vi "Send Perform Action on Target.vi"(7 "Message Priority (Normal)":T1=enum."Normal", 8 "error in":errorcluster, 9 "Point dent":string, 10 "Input":variant, 11 "Message Enqueuer":refnum<class "Message Enqueuer.lvclass">) -> (0 "error out":errorcluster, 2 "Output":variant, 3 "Message Enqueuer out":refnum<class "Message Enqueuer.lvclass">)   [LabVIEW 2023, in "IStudy Actor.lvlib" / "Perform Action on Target Msg.lvclass"]
doc: "This VI sends the message to an actor."
uses:
  Perform Action on Target Msg.lvclass
  Perform Action on Target Msg.lvclass/Perform Action on Target Msg.ctl
  DS-Reply-Msg/DS Reply Msg/DS Reply Msg.lvclass
  D:/git/DS-Reply-Msg/DS Reply Msg/DS Reply Msg.lvclass
  C:/Program Files/National Instruments/LabVIEW 2023/vi.lib/ActorFramework/Message/Message.lvclass
  D:/git/HAL/HAL GOOP4/Study/Study Actor/IStudy Actor Messages/Perform Action on Target Msg/Perform Action on Target Msg.lvclass
  <vilib>/ActorFramework/Message Enqueuer/Message Enqueuer.lvclass
  <vilib>/ActorFramework/Message Enqueuer/Message Priority.ctl
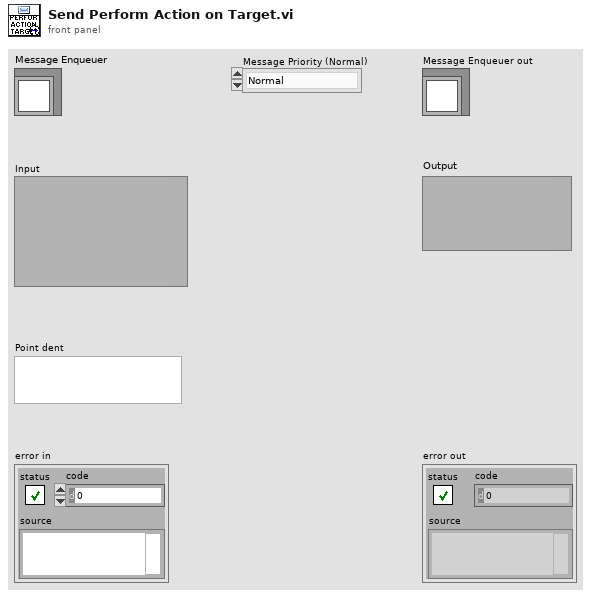
[diagram p1: front panel]
types:
  T1 = typedef "Actor Framework.lvlib/Message Enqueuer.lvclass/Message Priority.ctl" = enum16{"Low", "Normal", "High"}
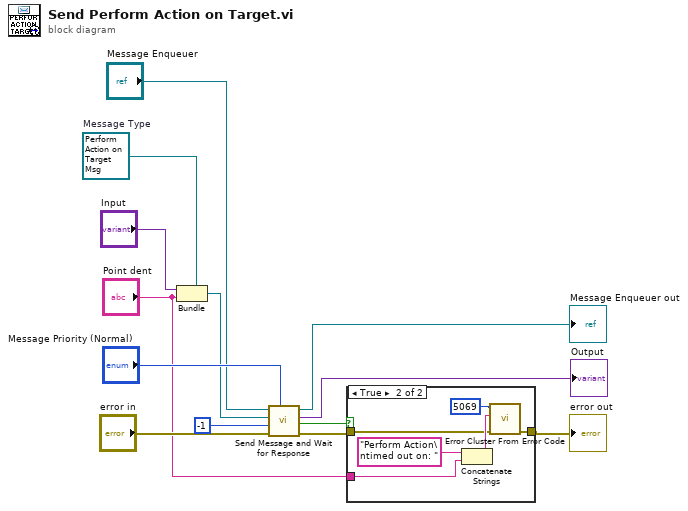
[diagram p0: block diagram]
diagram:
  w8 = refnum<class "Perform Action on Target Msg.lvclass"> refnum  # Message Type
  n1 = Bundle(cluster=w8, "Input", "Point dent") -> (w9:refnum<class "Perform Action on Target Msg.lvclass">)
  n2 = call "Send Message and Wait for Response.vi"("Message Priority (Normal)"="Message Priority (Normal)", "error in"="error in", "timeout in ms (-1)"=-1, "Original Message"=w9, "Message Enqueuer in"="Message Enqueuer") -> ("error out"=w4:errorcluster, "timed out?"=w5:bool, "Reply"=→"Output":variant, "Message Enqueuer out"=→"Message Enqueuer out":refnum<class "Message Enqueuer.lvclass">)  [unwired: 3 in]
  n3 = case shown="True" w5 {
    tunnel: w4 -> [w14 w15]
    tunnel: [w14 w20] -> w3
    tunnel: "Point dent" -> [_ w17]
    frame False {
    }
    frame True {
      n4 = Concatenate Strings("Perform Action\ntimed out on: ", w17) -> (w16:string)
      n5 = call <vilib>:"Error Cluster From Error Code.vi"("error in (no error)"=w15, "error message (\"\")"=w16, "error code (0)"=5069) -> ("error out"=w20:errorcluster)  [unwired: 6 in]
    }
  }
  "error out" <- w3
